vi "Choreo_TrajectoryDifferential_GetEvents.vi"(9 "eventName":string, 11 "ChoreoTrajectoryDifferential":T2) -> (3 "events":T1[](array[typedef]))   [LabVIEW 2019, in "ChoreoLib.lvlib"]
doc: "Returns a list of all events with the given name in the trajectory.\n \nInputs: \n -- ChoreoTrajectoryDifferential - cluster - data cluster for this trajectory \n -- eventName - string - The name of the event.\n\nOutputs: \n -- Events - cluster array - A list of all events with the given name in the trajectory, if no events are found, an empty list is returned."
uses:
  ChoreoLib.lvlib
  TypeDef/ChoreoTrajectoryDifferential.ctl
  TypeDef/ChoreoDifferentialSample.ctl
  TypeDef/ChoreoEventMarker.ctl
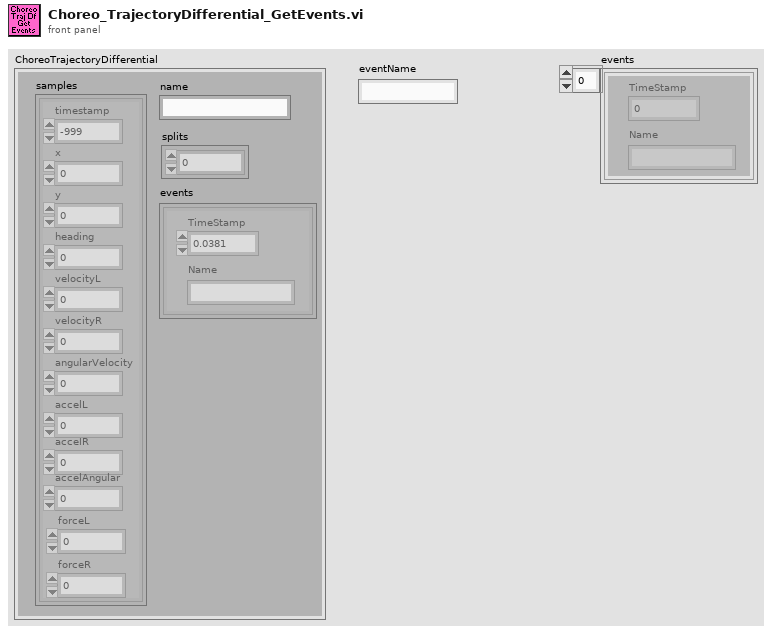
[diagram p1: front panel]
types:
  T1 = typedef "ChoreoLib.lvlib/ChoreoEventMarker.ctl" = cluster{"TimeStamp":dbl, "Name":string}
  T2 = typedef "ChoreoLib.lvlib/ChoreoTrajectoryDifferential.ctl" = cluster{"name":string, "samples":T3[], "splits":i32[], "events":T1[]}
  T3 = typedef "ChoreoLib.lvlib/ChoreoDifferentialSample.ctl" = cluster{"timestamp":dbl, "x":dbl, "y":dbl, "heading":dbl, "velocityL":dbl, "velocityR":dbl, "angularVelocity":dbl, "accelL":dbl, "accelR":dbl, "accelAngular":dbl, "forceL":dbl, "forceR":dbl}
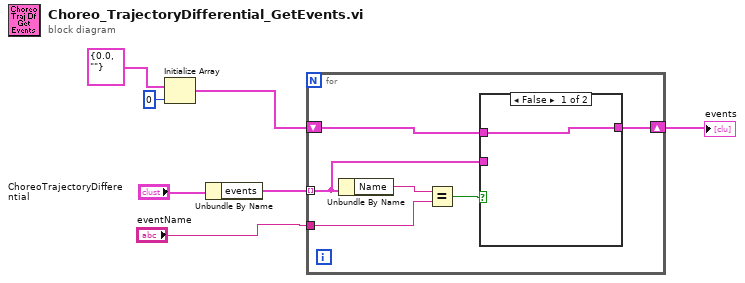
[diagram p0: block diagram]
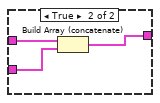
[diagram p2: hidden frame]
diagram:
  n1 = Initialize Array(T1 {"TimeStamp"=0.0, "Name"=""} ("ChoreoEvent"), 0 ("dimension size")) -> (w2:T1[])
  n2 = Unbundle By Name("ChoreoTrajectoryDifferential") -> ("events"=w6:T1[])
  n3 = for {
    tunnel: w6 -> [w9] mode=indexing
    tunnel: "eventName" -> [w12]
    shift-right: [w8] -> w1
    shift-left: w2 -> [w10]
    n4 = Unbundle By Name(w9) -> ("Name"=w13:string)
    n5 = Equal?(x=w13, y=w12) -> (x = y?=w11:bool)
    n6 = case shown="False" w11 {
      tunnel: w10 -> [w14 w17]
      tunnel: w9 -> [_ w16]
      tunnel: [w14 w15] -> w8
      frame False {
      }
      frame True {
        n7 = Build Array (concatenate)(w17, w16) -> (w15:T1[])
      }
    }
  }
  "events" <- w1
